vi "NCS_AmpPh.vi"(8 "IQ":cdb[](array[numeric]), 9 "data":cdb[][](array[numeric]), 10 "Sampling Rate":i32=500, 11 "Coerced Rx IQ Rate":dbl) -> (0 "Phase DownSampled":dbl[](array[numeric]), 1 "Amp DownSampled":dbl[](array[numeric]), 2 "Phase":dbl[](array[numeric]), 3 "Amplitude":dbl[](array[numeric]), 5 "x/y":dbl)   [LabVIEW 2016]
uses:
  <vilib>/Analysis/coordinate.llb/Wrap Angle (array).vi
  <vilib>/Analysis/3filter.llb/Butterworth Filter (DBL).vi
  <vilib>/Analysis/NI_AALBase.lvlib
  <vilib>/Analysis/NI_AALPro.lvlib
  <vilib>/Analysis/NI_AAL_Angle.lvlib
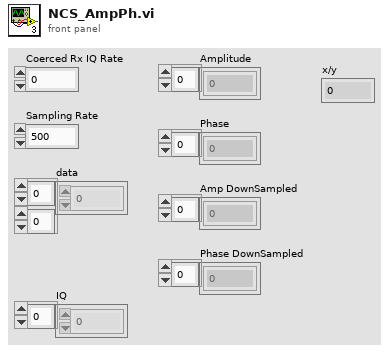
[diagram p1: front panel]
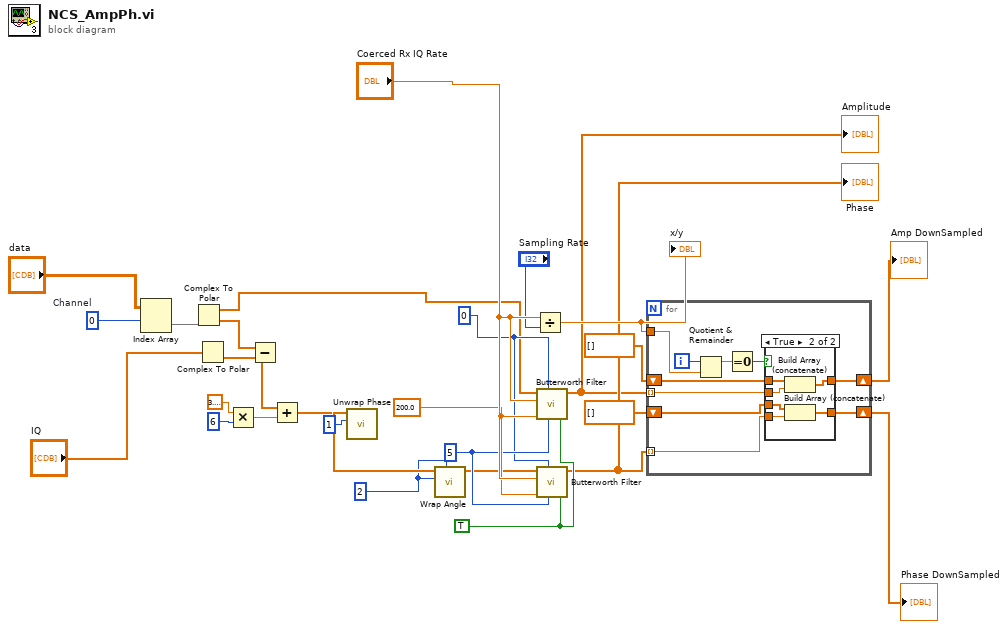
[diagram p0: block diagram]
diagram:
  w5 = 0  # Channel
  w23 = 5 ("order1")
  w27 = 200.0 ("Low-Pass Freq")
  w18 = 2 ("y")
  w24 = TRUE
  w22 = 0
  n1 = Index Array(array="data", index (row)=w5) -> (element=w3:cdb[])  [unwired: 1 in]
  n2 = Complex To Polar(r * e^(i*theta)=w3) -> (r=w9:dbl[], theta=w20:dbl[])
  n3 = Complex To Polar(r * e^(i*theta)="IQ") -> (theta=w14:dbl[])  [unwired: 1 out]
  n4 = Multiply(x=3.141592653589793, y=6) -> (x*y=w13:dbl)
  n5 = Subtract(x=w20, y=w14) -> (x-y=w16:dbl[])
  n6 = Add(x=w16, y=w13) -> (x+y=w17:dbl[])
  n7 = call <vilib>:"Unwrap Phase.vi"("phase unit"=1 ("y"), "Phase"=w17) -> ("Unwrapped Phase"=w19:dbl[])  [unwired: 8 in, 1 out]
  n8 = call-poly <vilib>:"Wrap Angle.vi"("angle units"=w18, "angle range"=w18, "Angle In"=w19) -> ("Angle Out"=w21:dbl[])  [unwired: 7 in, 1 out]
  n9 = Divide(x="Coerced Rx IQ Rate", y="Sampling Rate") -> (x/y=w8:dbl)
  "x/y" <- w8
  n10 = call-poly <vilib>:"Butterworth Filter.vi"("init/cont (init:F)"=w24, "order"=w23, "filter type"=w22, "low cutoff freq: fl"=w27, "sampling freq: fs"="Coerced Rx IQ Rate", "X"=w9) -> ("Filtered X"=w1:dbl[])  [unwired: 2 in, 1 out]
  "Amplitude" <- w1
  n11 = call-poly <vilib>:"Butterworth Filter.vi"("init/cont (init:F)"=w24, "order"=w23, "filter type"=w22, "low cutoff freq: fl"=w27, "sampling freq: fs"="Coerced Rx IQ Rate", "X"=w21) -> ("Filtered X"=w2:dbl[])  [unwired: 2 in, 1 out]
  "Phase" <- w2
  n12 = for {
    tunnel: w1 -> [w39] mode=indexing
    shift-right: [w37] -> w28
    shift-left: dbl[] [] -> [w38]
    tunnel: w8 -> [w33]
    shift-right: [w31] -> w26
    shift-left: dbl[] [] -> [w32]
    tunnel: w2 -> [w30] mode=indexing
    i -> [w36]
    n13 = Quotient & Remainder(x=w36, y=w33) -> (x-y*floor(x/y)=w34:dbl)  [unwired: 1 out]
    n14 = Equal To 0?(x=w34) -> (x = 0?=w35:bool)
    n15 = case shown="True" w35 {
      tunnel: w39 -> [_ w47]
      tunnel: w38 -> [w41 w46]
      tunnel: [w41 w45] -> w37
      tunnel: w32 -> [w40 w44]
      tunnel: [w40 w43] -> w31
      tunnel: w30 -> [_ w42]
      frame False {
      }
      frame True {
        n16 = Build Array (concatenate)(w46, w47) -> (w45:dbl[])
        n17 = Build Array (concatenate)(w44, w42) -> (w43:dbl[])
      }
    }
  }
  "Amp DownSampled" <- w28
  "Phase DownSampled" <- w26
